vi "SRV_Manage Window Sizes.vi"(0 "Sensor View ref":refnum<vi>, 1 "Vista or Later?":bool, 5 "Main Controller ref":refnum<vi>, 9 "Expand-Collapse":bool, 11 "error in (no error)":errorcluster, 13 "Update Main Controller Window Size (T)":bool=TRUE) -> (15 "error out":errorcluster)   [LabVIEW 2014]
uses:
  <vilib>/Utility/miscctls.llb/LVRectTypeDef.ctl
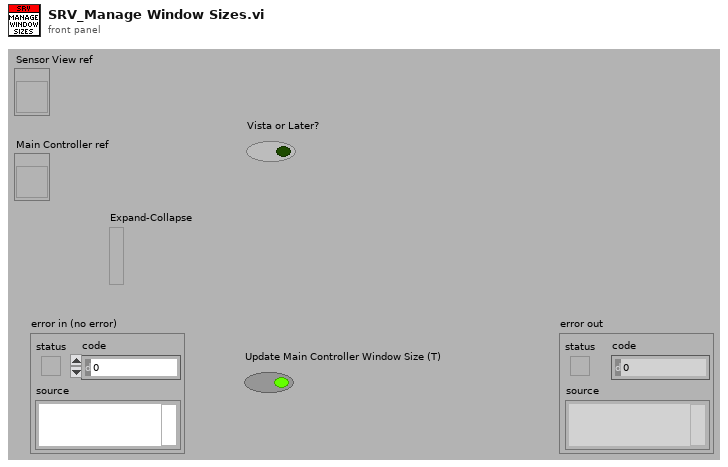
[diagram p1: front panel]
types:
  T1 = enum32{"Invalid", "Standard", "Closed", "Hidden", "Minimized", "Maximized"}
  T2 = typedef "LVRectTypeDef.ctl" = cluster{"Left":i16, "Top":i16, "Right":i16, "Bottom":i16}
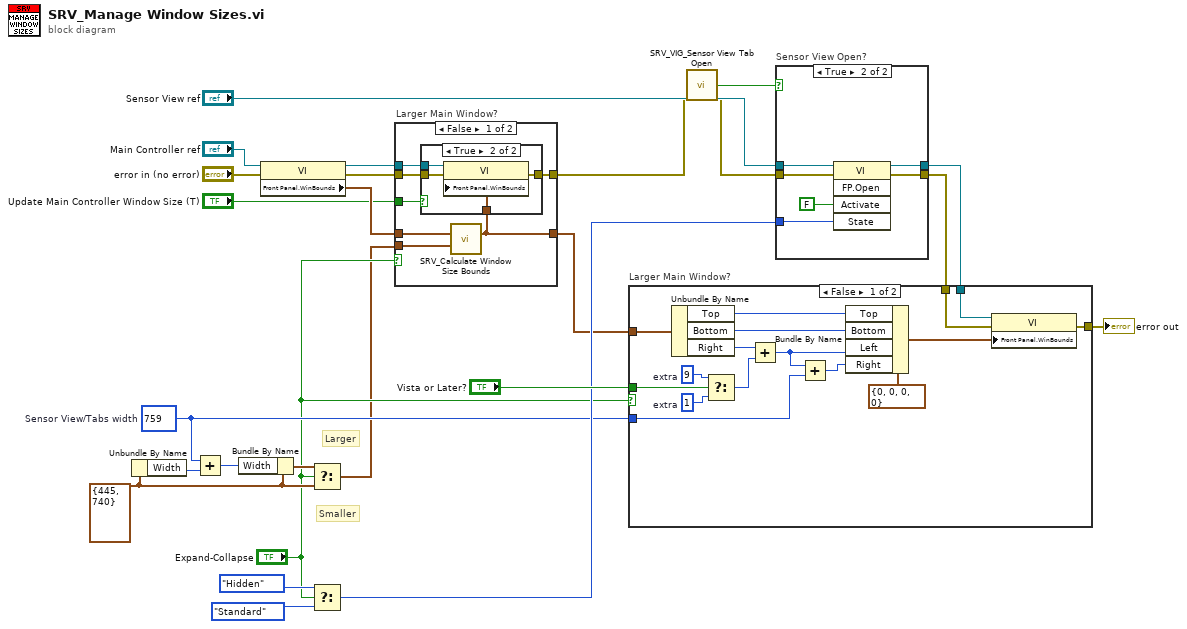
[diagram p0: block diagram]
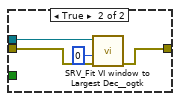
[diagram p5: hidden frame]
diagram:
  w12 = i16 759  # Sensor View/Tabs width
  w14 = cluster{"Width":i16, "Height":i16} {"Width"=445, "Height"=740} ("FP Width-Height")
  # "Larger"
  # "Smaller"
  n1 = Unbundle By Name(w14) -> ("Width"=w13:i16)
  n2 = Add(x=w12, y=w13) -> (x+y=w11:i16)
  n3 = Bundle By Name(cluster=w14, "Width"=w11) -> (w10:cluster{"Width":i16, "Height":i16})
  n4 = property class="VI"(reference="Main Controller ref", error in="error in (no error)") -> (reference out=w21:refnum<vi>, error out=w22:errorcluster, "Front Panel.WinBounds"=w3:T2)
  n5 = Select(t=w10, s="Expand-Collapse", f=w14) -> (s? t:f=w2:cluster{"Width":i16, "Height":i16})
  n6 = Select(t=T1."Hidden" ("State"), s="Expand-Collapse", f=T1."Standard" ("State")) -> (s? t:f=w15:T1)
  n7 = case "Larger Main Window?" shown="False" "Expand-Collapse" {
    tunnel: w22 -> [w32 w39]
    tunnel: w21 -> [w31 w40]
    tunnel: [w30 w38] -> w19
    tunnel: [w29 _] -> w4
    tunnel: w3 -> [w28 _]
    tunnel: w2 -> [w27 _]
    tunnel: "Update Main Controller Window Size (T)" -> [w26 _]
    frame False {
      n8 = call "SRV_Calculate Window Size Bounds.vi"("FP Window Bounds"=w28, "FP Width-Height"=w27) -> ("FP Window Bounds out"=w29:T2)  [unwired: 13 in]
      n9 = case shown="True" w26 {
        tunnel: w32 -> [w33 w37]
        tunnel: w31 -> [_ w36]
        tunnel: [w33 w35] -> w30
        tunnel: w29 -> [_ w34]
        frame False {
        }
        frame True {
          n10 = property class="VI"(reference=w36, error in=w37, "Front Panel.WinBounds"=w34) -> (error out=w35:errorcluster)  [unwired: 1 out]
        }
      }
    }
    frame True {
      n11 = call "SRV_Fit VI window to Largest Dec__ogtk.vi"("error in (no error)"=w39, "border spacing (2 px)"=0, "VI Ref (calling VI)"=w40) -> ("error out"=w38:errorcluster)  [unwired: 3 in, 1 out]
    }
  }
  n12 = call "SRV_VIG_Sensor View Tab Open.vi"("error in (no error)"=w19) -> ("Sensor View Tab Open?"=w6:bool, "error out"=w18:errorcluster)  [unwired: 13 in]
  n13 = case "Sensor View Open?" shown="True" w6 {
    tunnel: "Sensor View ref" -> [w43 w49]
    tunnel: w18 -> [w42 w48]
    tunnel: w15 -> [_ w47]
    tunnel: [w42 w46] -> w9
    tunnel: [w43 w45] -> w7
    frame False {
    }
    frame True {
      n14 = invoke class="VI" method="FP.Open"(reference=w49, error in=w48, "Activate"=FALSE ("Activate?"), "State"=w47) -> (reference out=w45:refnum<vi>, error out=w46:errorcluster)  [unwired: 1 in, 3 out]
    }
  }
  n15 = case "Larger Main Window?" shown="False" "Expand-Collapse" {
    tunnel: w4 -> [w65 _]
    tunnel: "Vista or Later?" -> [w64 _]
    tunnel: w12 -> [w63 _]
    tunnel: w9 -> [w62 w66]
    tunnel: [w61 w66] -> w8
    tunnel: w7 -> [w60 _]
    frame False {
      w51 = i16 9  # extra
      w52 = i16 1  # extra
      n16 = Unbundle By Name(w65) -> ("Top"=w55:i16, "Bottom"=w54:i16, "Right"=w57:i16)
      n17 = Select(t=w51, s=w64, f=w52) -> (s? t:f=w50:i16)
      n18 = Add(x=w57, y=w50) -> (x+y=w58:i16)
      n19 = Add(x=w58, y=w63) -> (x+y=w56:i16)
      n20 = Bundle By Name(cluster=T2 {"Left"=0, "Top"=0, "Right"=0, "Bottom"=0} ("Front Panel Window:Window Bounds"), "Top"=w55, "Bottom"=w54, "Left"=w58, "Right"=w56) -> (w59:T2)
      n21 = property class="VI"(reference=w60, error in=w62, "Front Panel.WinBounds"=w59) -> (error out=w61:errorcluster)  [unwired: 1 out]
    }
    frame True {
    }
  }
  "error out" <- w8
